vi "SetDisplayMeasureFunction.vi"(7 "SMU":T2, 8 "Error In":errorcluster, 10 "Display Function":T1, 11 "Keithley 2602 In":refnum<visa-resource-name>) -> (0 "Error Out":errorcluster, 3 "Keithley 2602 Out":refnum<visa-resource-name>)   [LabVIEW 2012, in "Keithley-2602.lvlib"]
uses:
  Keithley-2602.lvlib
  Controls/SMU.ctl
  Controls/DisplayFunction.ctl
panel:
  out "Command":string
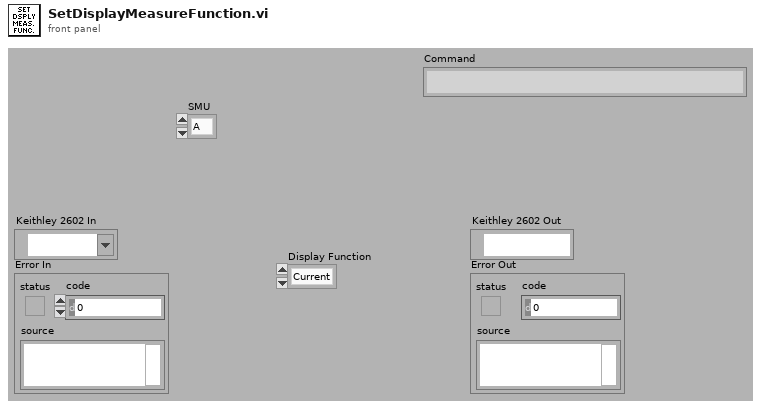
[diagram p1: front panel]
types:
  T1 = typedef "Keithley-2602.lvlib/DisplayFunction.ctl" = enum16{"Current", "Voltage", "Resistance", "Power"}
  T2 = typedef "Keithley-2602.lvlib/SMU.ctl" = enum16{"A", "B"}
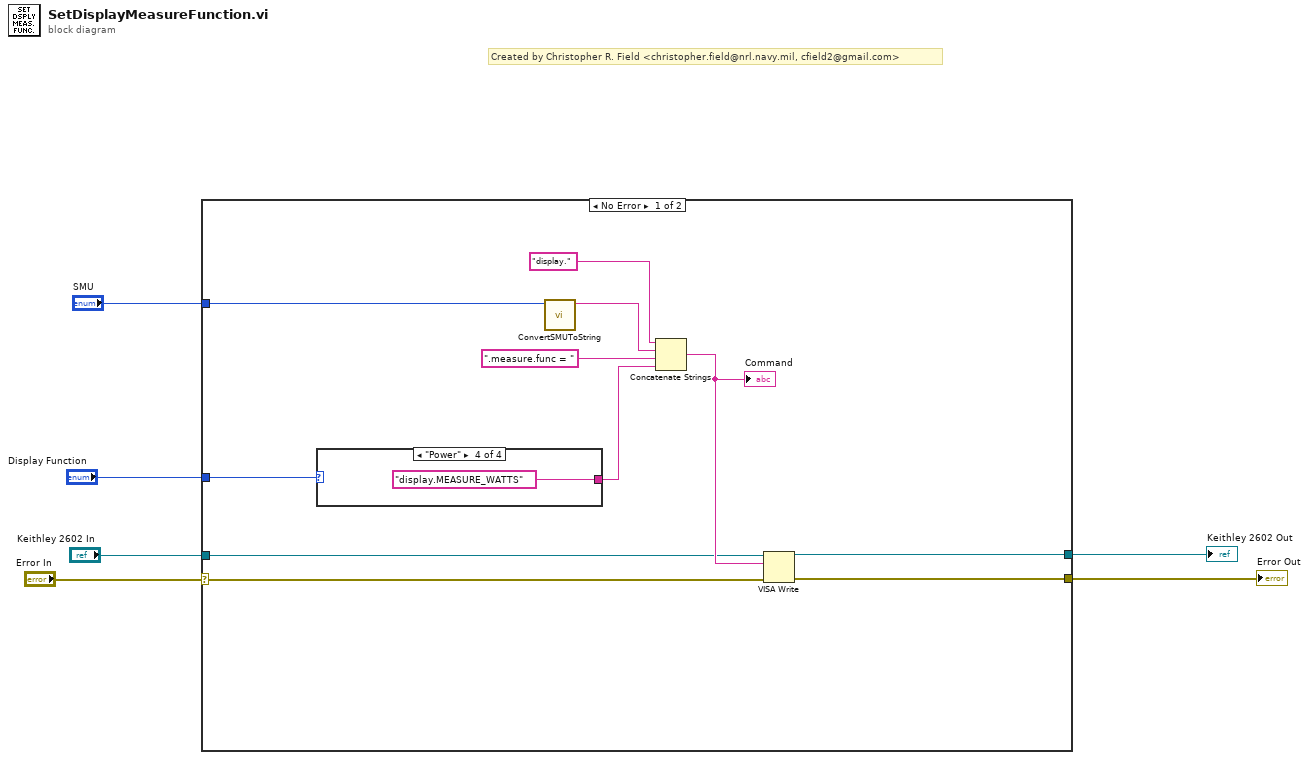
[diagram p0: block diagram]
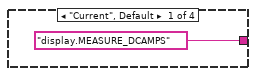
[diagram p2: hidden frame]
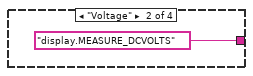
[diagram p3: hidden frame]
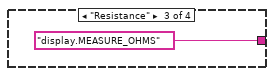
[diagram p4: hidden frame]
diagram:
  # "Created by Christopher R. Field <christopher.field@nrl.navy.mil, cfield2@gmail.com>"
  n1 = case shown="No Error" "Error In" {
    selector: "Error In" -> [w7 w22]
    tunnel: "Keithley 2602 In" -> [w16 w23]
    tunnel: [w15 w23] -> w5
    tunnel: [w14 w22] -> w4
    tunnel: "Display Function" -> [w9 _]
    tunnel: "SMU" -> [w8 _]
    frame No Error {
      n2 = case shown="\"Power\"" w9 {
        tunnel: ["display.MEASURE_DCAMPS" "display.MEASURE_DCVOLTS" "display.MEASURE_OHMS" "display.MEASURE_WATTS"] -> w10
        frame "Current", Default {
        }
        frame "Voltage" {
        }
        frame "Resistance" {
        }
        frame "Power" {
        }
      }
      n3 = call "ConvertSMUToString.vi"("SMU"=w8) -> ("Channel"=w12:string)  [unwired: 10 in]
      n4 = Concatenate Strings("display.", w12, ".measure.func = " ("string"), w10) -> (w17:string)
      "Command" <- w17
      n5 = VISA Write(VISA resource name=w16, write buffer=w17, error in (no error)=w7) -> (VISA resource name out=w15:refnum<visa-resource-name>, error out=w14:errorcluster)  [unwired: 1 out]
    }
    frame Error {
    }
  }
  "Keithley 2602 Out" <- w5
  "Error Out" <- w4
